vi "Main.vi"() -> ()   [LabVIEW 2019]
uses:
  <vilib>/Utility/miscctls.llb/LVPositionTypeDef.ctl
  State.ctl
panel:
  out "Ball":bool
  in  "Coefficient of restitution":dbl=0.8 format="%#_13g"
  out "State":T1
  in  "Stop":bool
  in  "Start":bool
  out "Position":T2
  out "Speed":dbl
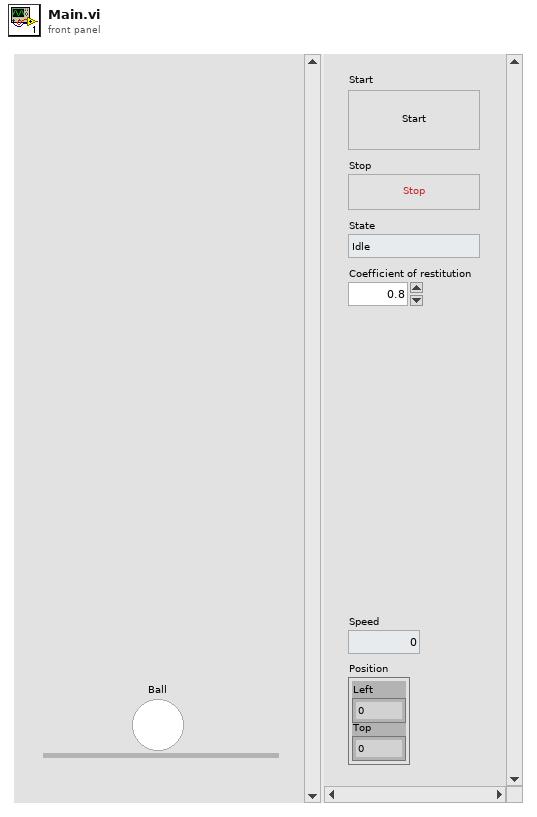
[diagram p1: front panel]
types:
  T1 = typedef "State.ctl" = enum16{"Idle", "Switch mode", "Falling", "Rising"}
  T2 = typedef "LVPositionTypeDef.ctl" = cluster{"Left":i32, "Top":i32}
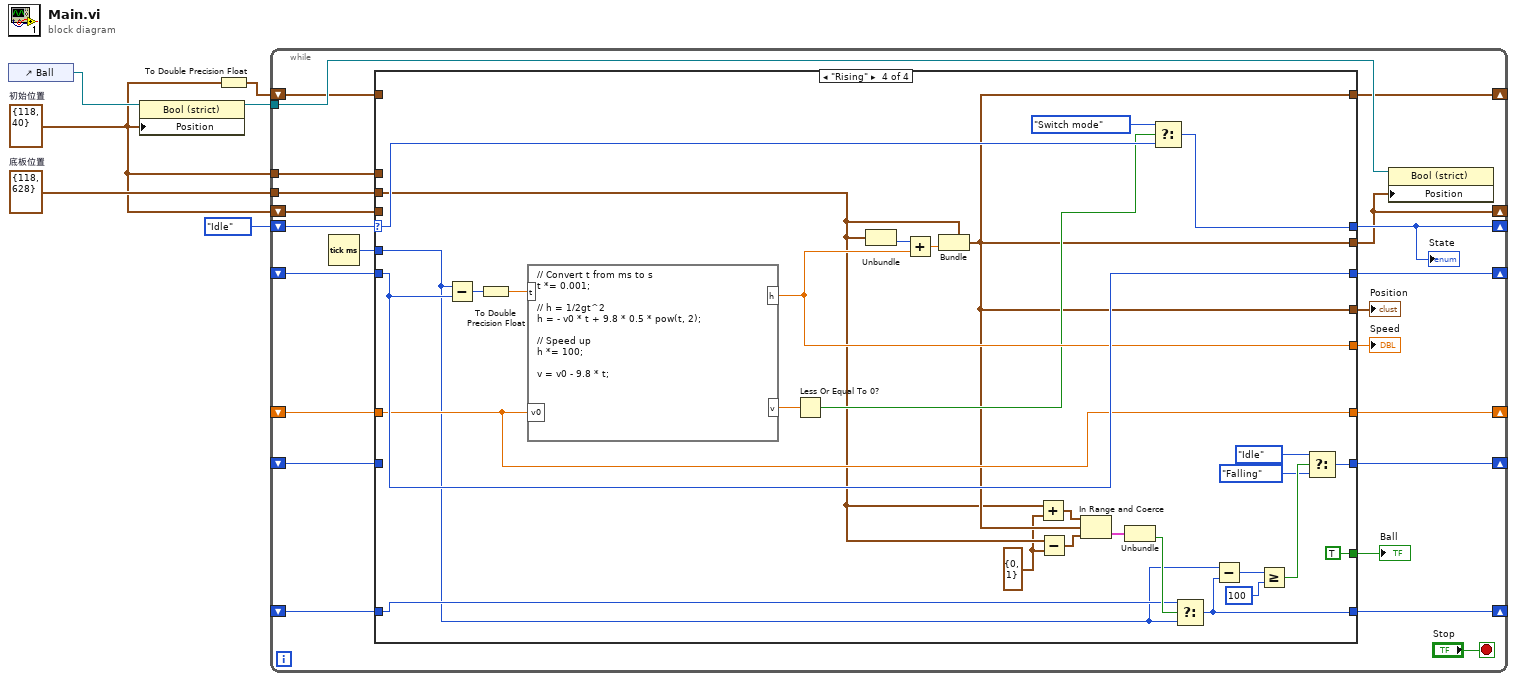
[diagram p0: block diagram]
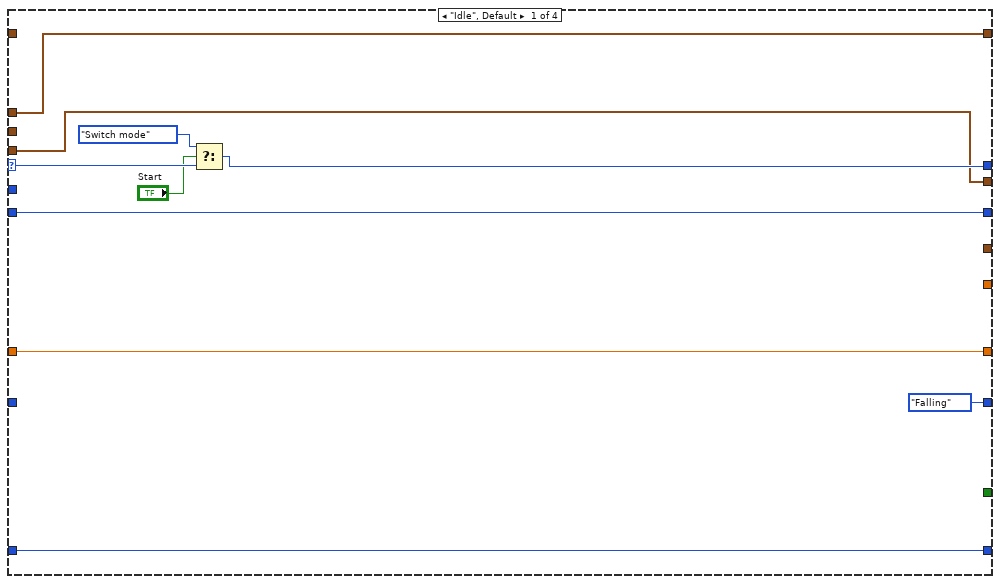
[diagram p2: hidden frame]
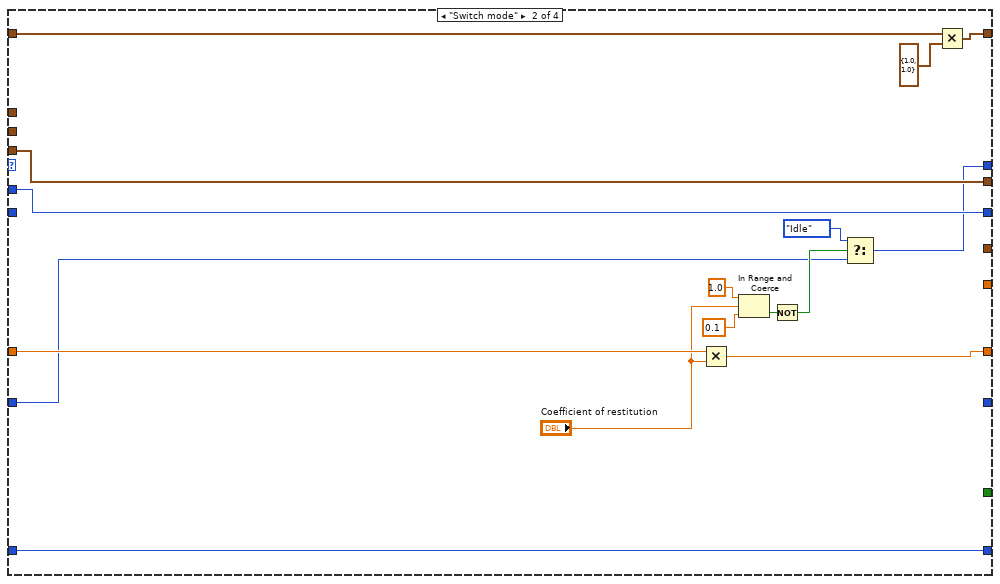
[diagram p3: hidden frame]
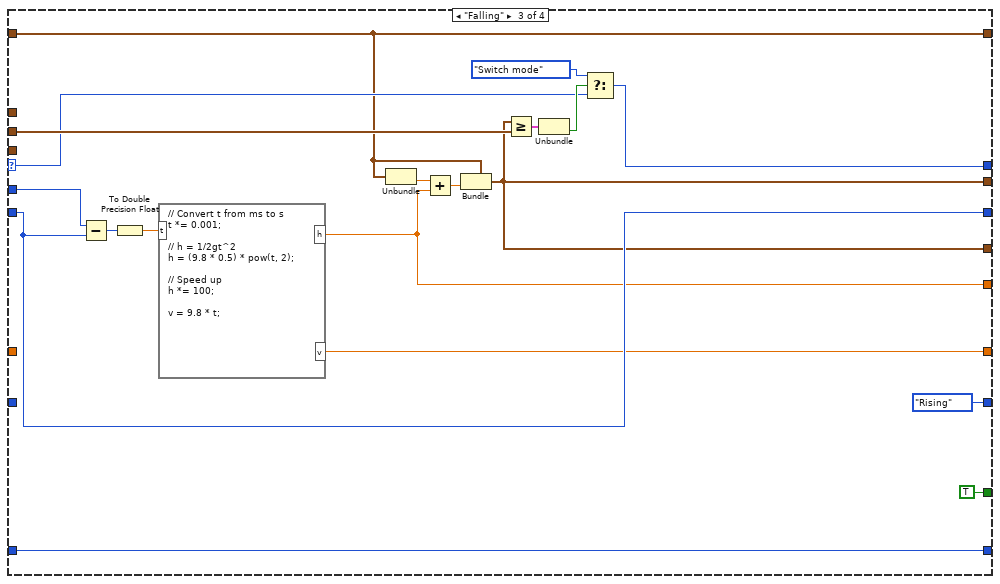
[diagram p4: hidden frame]
diagram:
  w5 = T2 {"Left"=118, "Top"=628}  # 底板位置
  w2 = T2 {"Left"=118, "Top"=40}  # 初始位置
  n1 = control-ref of="Ball"() -> (w3:refnum<vi>)
  n2 = property class="Bool (strict)"(reference=w3, "Position"=w2) -> (reference out=w6:refnum<vi>)  [unwired: 1 in, 1 out]
  n3 = To Double Precision Float(number=w2) -> (double precision float=w1:cluster{"Left":dbl, "Top":dbl})
  n4 = while {
    tunnel: w6 -> [w21]
    tunnel: w2 -> [w28]
    tunnel: w5 -> [w27]
    shift-right: [w25] -> _
    shift-left: State."Idle" -> [w26]
    shift-right: [w23] -> _
    shift-left: _ -> [w22]
    shift-right: [w19] -> _
    shift-left: _ -> [w18]
    shift-right: [w15] -> _
    shift-left: _ -> [w14]
    shift-right: [w12] -> _
    shift-left: w2 -> [w20]
    shift-right: [w11] -> _
    shift-left: w1 -> [w10]
    shift-right: [w9] -> _
    shift-left: _ -> [w8]
    stop <- "Stop" stop-if-true
    n5 = Tick Count (ms)() -> (millisecond timer value=w13:u32)
    n6 = case shown="\"Rising\"" w26 {
      selector: w26 -> [w38 _ w65 w97]
      tunnel: w28 -> [w29 _ _ _]
      tunnel: w27 -> [_ _ w69 w87]
      tunnel: [w35 w39 w64 w96] -> w25
      tunnel: [w34 w54 w67 w98] -> w23
      tunnel: w22 -> [w34 _ w67 w98]
      tunnel: [w31 w53 w61 w90] -> w12
      tunnel: w20 -> [w31 w53 _ _]
      tunnel: [State."Falling" ("t") _ State."Rising" ("t") w77] -> w19
      tunnel: w18 -> [_ w40 _ _]
      tunnel: [_ _ w61 w90] -> w17
      tunnel: [_ _ w60 w94] -> w16
      tunnel: [w32 w48 w59 w93] -> w15
      tunnel: w14 -> [w32 w49 _ w93]
      tunnel: w13 -> [_ w54 w58 w82]
      tunnel: [w29 w50 w57 w90] -> w11
      tunnel: w10 -> [_ w51 w57 _]
      tunnel: [w30 w43 w56 w81] -> w9
      tunnel: w8 -> [w30 w43 w56 w83]
      tunnel: [_ _ TRUE ("Ball") TRUE ("Ball")] -> w7
      frame "Idle", Default {
        n7 = Select(t=State."Switch mode", s="Start", f=w38) -> (s? t:f=w35:T1)
      }
      frame "Switch mode" {
        n8 = Multiply(x=w49, y="Coefficient of restitution") -> (x*y=w48:dbl)
        n9 = In Range and Coerce(upper limit=1.0 ("lower limit"), x="Coefficient of restitution", lower limit=0.1) -> (In Range?=w44:bool)  [unwired: 1 out]
        n10 = Not(x=w44) -> (.not. x?=w42:bool)
        n11 = Select(t=State."Idle", s=w42, f=w40) -> (s? t:f=w39:T1)
        n12 = Multiply(x=w51, y=cluster{dbl, dbl} {1.0, 1.0}) -> (x*y=w50:cluster{dbl, dbl})
      }
      frame "Falling" {
        n13 = Subtract(x=w58, y=w67) -> (x-y=w72:u32)
        n14 = To Double Precision Float(number=w72) -> (double precision float=w71:dbl)
        n15 = formula code="// Convert t from ms to s\nt *= 0.001;\n\n// h = 1/2gt^2\nh = (9.8 * 0.5) * pow(t, 2);\n\n// Speed up\nh *= 100;\n\nv = 9.8 * t;"("t"=w71) -> ("h"=w60:dbl, "v"=w59:dbl)
        n16 = Unbundle(w57) -> ("Top"=w73:dbl)  [unwired: 1 out]
        n17 = Add(x=w73, y=w60) -> (x+y=w70:dbl)
        n18 = Bundle(cluster=w57, "Top"=w70) -> (w61:cluster{"Left":dbl, "Top":dbl})  [unwired: 1 in]
        n19 = Greater Or Equal?(x=w61, y=w69) -> (x >= y?=w68:cluster{"Left":bool, "Top":bool})
        n20 = Unbundle(w68) -> ("Top"=w66:bool)  [unwired: 1 out]
        n21 = Select(t=State."Switch mode", s=w66, f=w65) -> (s? t:f=w64:T1)
      }
      frame "Rising" {
        w86 = T2 {"Left"=0, "Top"=1} ("y")
        n22 = Subtract(x=w82, y=w98) -> (x-y=w101:u32)
        n23 = To Double Precision Float(number=w101) -> (double precision float=w100:dbl)
        n24 = formula code="// Convert t from ms to s\nt *= 0.001;\n\n// h = 1/2gt^2\nh = - v0 * t + 9.8 * 0.5 * pow(t, 2);\n\n// Speed up\nh *= 100;\n\nv = v0 - 9.8 * t;"("t"=w100, "v0"=w93) -> ("h"=w94:dbl, "v"=w92:dbl)
        n25 = Less Or Equal To 0?(x=w92) -> (x <= 0?=w91:bool)
        n26 = Unbundle(w87) -> ("Top"=w102:i32)  [unwired: 1 out]
        n27 = Add(x=w102, y=w94) -> (x+y=w99:dbl)
        n28 = Bundle(cluster=w87, "Top"=w99) -> (w90:T2)  [unwired: 1 in]
        n29 = Add(x=w87, y=w86) -> (x+y=w89:T2)
        n30 = Subtract(x=w87, y=w86) -> (x-y=w88:T2)
        n31 = In Range and Coerce(upper limit=w89, x=w90, lower limit=w88) -> (In Range?=w85:cluster{"Left":bool, "Top":bool})  [unwired: 1 out]
        n32 = Unbundle(w85) -> ("Top"=w84:bool)  [unwired: 1 out]
        n33 = Select(t=State."Switch mode", s=w91, f=w97) -> (s? t:f=w96:T1)
        n34 = Select(t=w83, s=w84, f=w82) -> (s? t:f=w81:u32)
        n35 = Subtract(x=w82, y=w81) -> (x-y=w80:u32)
        n36 = Greater Or Equal?(x=w80, y=u32 100) -> (x >= y?=w78:bool)
        n37 = Select(t=State."Idle", s=w78, f=State."Falling" ("t")) -> (s? t:f=w77:T1)
      }
    }
    "Position" <- w17
    "Speed" <- w16
    "State" <- w25
    "Ball" <- w7
    n38 = property class="Bool (strict)"(reference=w21, "Position"=w12) -> ()  [unwired: 1 in, 2 out]
  }
